vi "crc_check.vi"(3 "input bit":i16[](array[numeric])) -> (0 "CRC valid":bool, 1 "splited":i16[](array[numeric]))   [LabVIEW 2014]
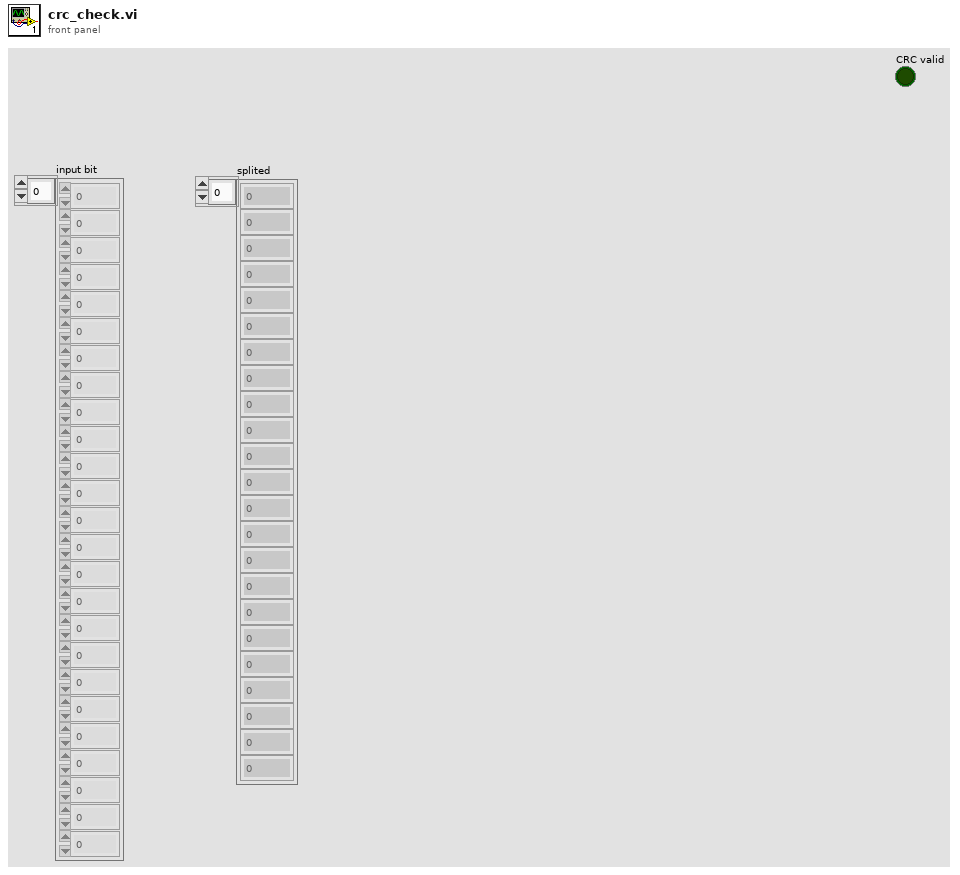
[diagram p1: front panel]
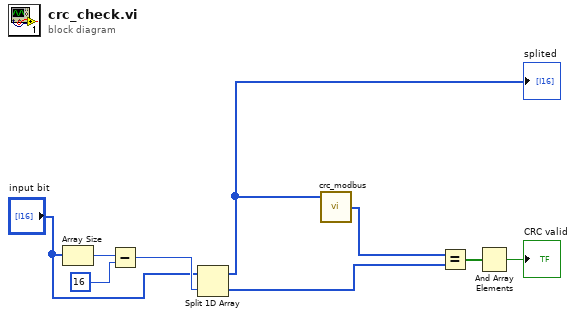
[diagram p0: block diagram]
diagram:
  n1 = Array Size(array="input bit") -> (size(s)=w9:i32)
  n2 = Subtract(x=w9, y=16 ("index")) -> (x-y=w6:i32)
  n3 = Split 1D Array(array="input bit", index=w6) -> (first subarray=w4:i16[], second subarray=w3:i16[])
  "splited" <- w4
  n4 = call "crc_modbus.vi"("input bit"=w4) -> ("crc"=w7:i16[])  [unwired: 3 in, 1 out]
  n5 = Equal?(x=w7, y=w3) -> (x = y?=w2:bool[])
  n6 = And Array Elements(Boolean array=w2) -> (logical AND=→"CRC valid":bool)
